vi "5302GetOscVolts.vi"(8 "error in (no error)":errorcluster, 11 "VISA Resource Name":refnum<visa-resource-name>) -> (0 "error out":errorcluster, 1 "data string":string, 2 "Osc Volts":dbl format="%.4f", 3 "VISA Resource Name Out":refnum<visa-resource-name>)   [LabVIEW 2015]
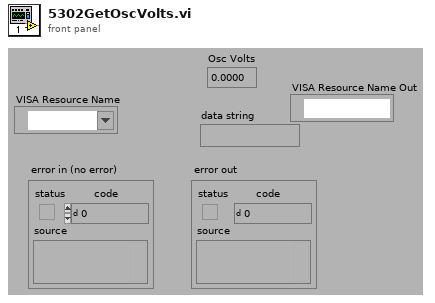
[diagram p1: front panel]
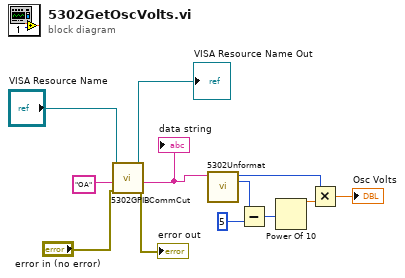
[diagram p0: block diagram]
diagram:
  n1 = call "5302GPIBCommCut.vi"("error in (no error)"="error in (no error)", "data string in"="OA" ("data string"), "VISA Resource Name"="VISA Resource Name") -> ("error out"=→"error out":errorcluster, "data string out"=w9:string, "VISA Resource Name Out"=→"VISA Resource Name Out":refnum<visa-resource-name>)  [unwired: 2 in, 4 out]
  "data string" <- w9
  n2 = call "5302Unformat.vi"("Data String"=w9) -> ("Numeric 2"=w3:i32, "Numeric 1"=w6:i32)  [unwired: 9 out]
  n3 = Subtract(x=w3, y=5) -> (x-y=w7:i32)
  n4 = Power Of 10(x=w7) -> (10^x=w5:dbl)
  n5 = Multiply(x=w6, y=w5) -> (x*y=→"Osc Volts":dbl)
